vi "set_command_position.vi"(8 "error in (no error)":errorcluster, 10 "command position":refnum<class "SpaceVector.lvclass">, 11 "DL090409StageScaffold.lvclass in":refnum<class "StageDL090409Scaffold.lvclass">) -> (0 "error out":errorcluster, 3 "DL090409StageScaffold.lvclass out":refnum<class "StageDL090409Scaffold.lvclass">)   [LabVIEW 2010, in "StageDL090409Scaffold.lvclass"]
uses:
  StageDL090409Scaffold.lvclass
  common/classes/SpaceVector/SpaceVector/SpaceVector.lvclass
  StageDL090409Scaffold.lvclass/StageDL090409Scaffold.ctl
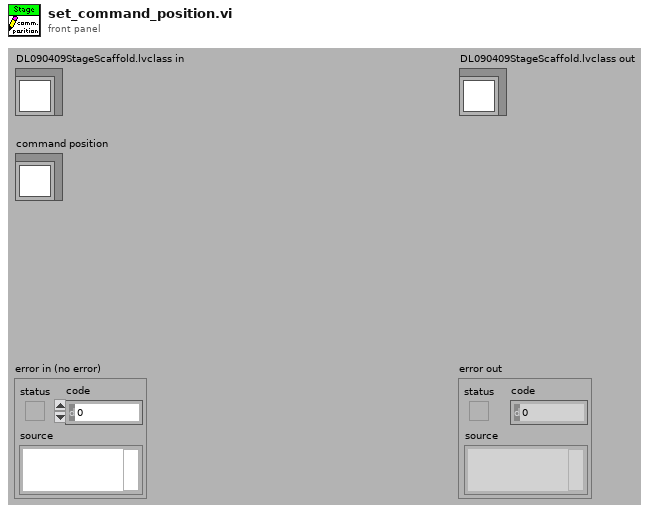
[diagram p1: front panel]
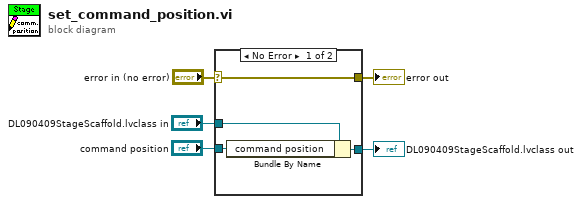
[diagram p0: block diagram]
diagram:
  n1 = case shown="No Error" "error in (no error)" {
    selector: "error in (no error)" -> [w9 w10]
    tunnel: [w9 w10] -> w4
    tunnel: [w7 w11] -> w2
    tunnel: "DL090409StageScaffold.lvclass in" -> [w8 w11]
    tunnel: "command position" -> [w6 _]
    frame No Error {
      n2 = Bundle By Name(cluster=w8, "command position"=w6) -> (w7:refnum<class "StageDL090409Scaffold.lvclass">)
    }
    frame Error {
    }
  }
  "error out" <- w4
  "DL090409StageScaffold.lvclass out" <- w2
